vi "Create CANBus Load Calculator.vi"(8 "error in (no error)":errorcluster, 10 "Calculation Period (ms)":u32=500, 11 "XNET Session":refnum<k21>) -> (0 "error out":errorcluster, 3 "CANBus Load Calculator":refnum<class "CANBus_Load_Calculator.lvclass">)   [LabVIEW 2018, in "NI-XNET Monitor Engine.lvlib" / "XNET-Bus-Load-Calculator.lvlib"]
uses:
  XNET-Bus-Load-Calculator.lvlib
  CANBus/CANBus_Load_Calculator.lvclass
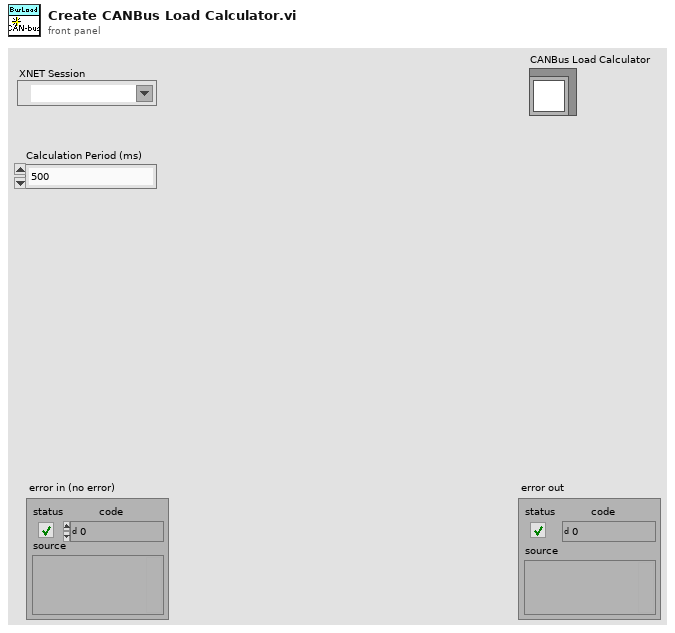
[diagram p1: front panel]
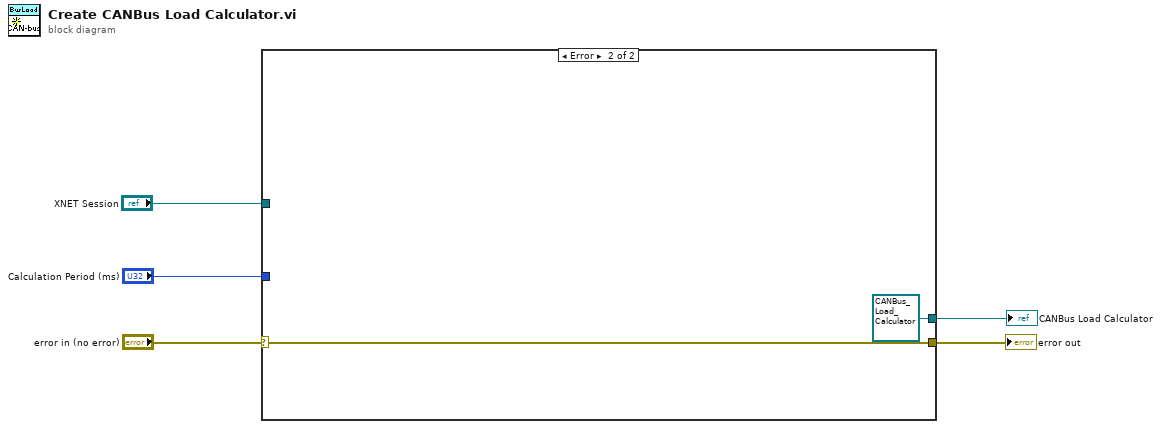
[diagram p0: block diagram]
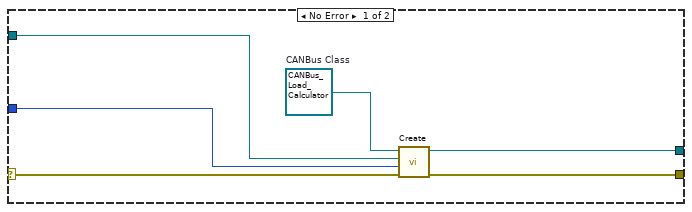
[diagram p2: hidden frame]
diagram:
  n1 = case shown="Error" "error in (no error)" {
    selector: "error in (no error)" -> [w10 w13]
    tunnel: [w9 w13] -> w4
    tunnel: "XNET Session" -> [w8 _]
    tunnel: "Calculation Period (ms)" -> [w7 _]
    tunnel: [w6 refnum<class "CANBus_Load_Calculator.lvclass"> refnum ("CANBus_Load_Calculator out")] -> w1
    frame No Error {
      w11 = refnum<class "CANBus_Load_Calculator.lvclass"> refnum  # CANBus Class
      n2 = call "Create.vi"("error in (no error)"=w10, "Calculation Period (ms)"=w7, "XNET Session"=w8, "CANBus_Load_Calculator in"=w11) -> ("error out"=w9:errorcluster, "CANBus_Load_Calculator out"=w6:refnum<class "CANBus_Load_Calculator.lvclass">)  [unwired: 6 in]
    }
    frame Error {
    }
  }
  "error out" <- w4
  "CANBus Load Calculator" <- w1
